vi "Load experiment header stats.vi"(11 "Funct data structure":bool) -> (2 "Experiment Header's Statistics":T1, 3 "Acquisition time unknown":bool)   [LabVIEW 2017]
uses:
  Typedefs/Test header stats cluster.ctl
  Globals/gl_Time series viewer globals.vi
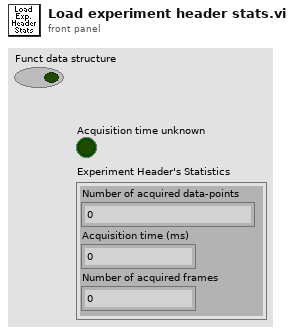
[diagram p1: front panel]
types:
  T1 = typedef "Test header stats cluster.ctl" = cluster{"Number of acquired data-points":dbl, "Acquisition time (ms)":dbl, "Number of acquired frames":dbl}
  T2 = typedef "Time series viewer refs.ctl" = cluster{"This VI":refnum<vi>, "Image control":refnum<vi>, "AVI Mode ind":refnum<vi>, "Play":refnum<vi>, "Stop":refnum<vi>, "Back":refnum<vi>, "Scrollbar":refnum<vi>, "Video length info":refnum<vi>, "Expected speed values":refnum<vi>, "Intensity":refnum<vi>, "Path":refnum<vi>, "Selection sliders":refnum<vi>, "Speed Graph ref":refnum<vi>, "Frame rate set (fps)":refnum<vi>, "Channel to load":refnum<vi>, "Number of rows to generate":refnum<vi>, "Colour":refnum<vi>}
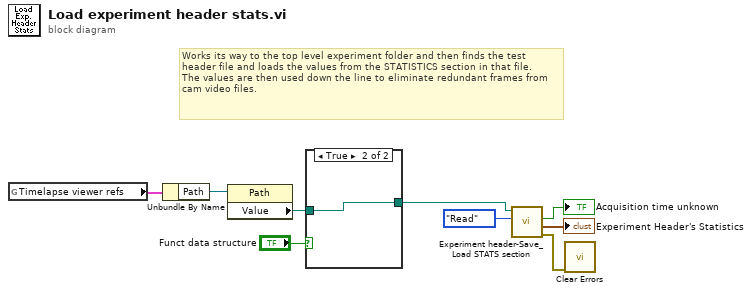
[diagram p0: block diagram]
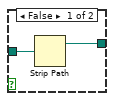
[diagram p2: hidden frame]
diagram:
  # "Works its way to the top level experiment folder and then finds the test header file and loads the values from the STATISTICS section in that file.\nThe values are then used down the line to eliminate redundant frames from cam video files."
  n1 = global read "gl_Time series viewer globals.vi" "Timelapse viewer refs"() -> (w4:T2)
  n2 = Unbundle By Name(w4) -> ("Path"=w5:refnum<vi>)
  n3 = property class="Path"(reference=w5) -> ("Value"=w6:path)  [unwired: 1 in, 2 out]
  n4 = case shown="True" "Funct data structure" {
    tunnel: w6 -> [w11 w12]
    tunnel: [w10 w12] -> w3
    frame False {
      n5 = Strip Path(path=w11) -> (stripped path=w10:path)  [unwired: 1 out]
    }
    frame True {
    }
  }
  n6 = call "Experiment header-Save_Load STATS section.vi"("Function"=enum16{"Write", "Read"}."Read", "Experiment folder path"=w3) -> ("error out"=w2:errorcluster, "Read values"=→"Experiment Header's Statistics":T1, "Acquisition time unknown"=→"Acquisition time unknown":bool)  [unwired: 7 in]
  n7 = call <vilib>:"Clear Errors.vi"("error in (no error)"=w2) -> ()  [unwired: 5 in, 2 out]
